vi "Write Basic CD Properties.vi"(8 "Error In":errorcluster, 10 "Main CD Properties":T1, 11 "Custom Device .NET Ref In":refnum<k24>) -> (0 "Error Out":errorcluster, 3 "Custom Device .NET Ref Out":refnum<k24>)   [LabVIEW 2015, in "VeriStand Custom Device XML Parser.lvlib"]
doc: "Sets the main properties of the custom device"
uses:
  VeriStand Custom Device XML Parser.lvlib
  NationalInstruments.VeriStand.XMLReader
  XML Controls/Main Custom Device Properties.ctl
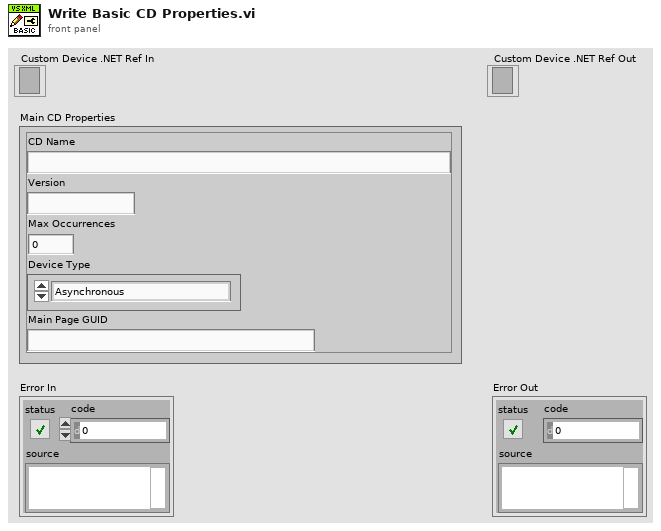
[diagram p1: front panel]
types:
  T1 = typedef "VeriStand Custom Device XML Parser.lvlib/Main Custom Device Properties.ctl" = cluster{"CD Name":string, "Version":string, "Max Occurrences":i32, "Device Type":enum16{"Asynchronous", "Inline HW Interface", "Inline Model Interface", "Inline Timing and Sync", "Asynchronous Timing and Sync"}, "Main Page GUID":string}
  T2 = enum16{"Asynchronous", "Inline HW Interface", "Inline Model Interface", "Inline Timing and Sync", "Asynchronous Timing and Sync"}
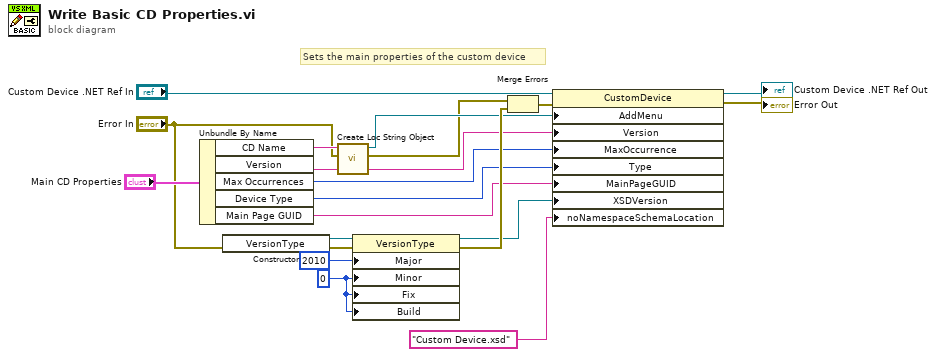
[diagram p0: block diagram]
diagram:
  w14 = u32 0 ("Major")
  # "Sets the main properties of the custom device"
  n1 = Unbundle By Name("Main CD Properties") -> ("CD Name"=w4:string, "Version"=w7:string, "Max Occurrences"=w8:i32, "Device Type"=w9:T2, "Main Page GUID"=w10:string)
  n2 = constructor class="VersionType"(error in="Error In") -> (reference out=w12:refnum<k24>, error out=w11:errorcluster)  [unwired: 2 in, 1 out]
  n3 = call "Create Loc String Object.vi"("Error In"="Error In", "String Input"=w4) -> ("Error Out"=w1:errorcluster, "Loc String .NET Ref"=w2:refnum<k24>)  [unwired: 8 in]
  n4 = property class="VersionType"(reference=w12, error in=w11, "Major"=u32 2010, "Minor"=w14, "Fix"=w14, "Build"=w14) -> (reference out=w15:refnum<k24>, error out=w16:errorcluster)
  n5 = Merge Errors(w1, w16) -> (w17:errorcluster)
  n6 = property class="CustomDevice"(reference="Custom Device .NET Ref In", error in=w17, "AddMenu"=w2, "Version"=w7, "MaxOccurrence"=w8, "Type"=w9, "MainPageGUID"=w10, "XSDVersion"=w15, "noNamespaceSchemaLocation"="Custom Device.xsd") -> (reference out=→"Custom Device .NET Ref Out":refnum<k24>, error out=→"Error Out":errorcluster)
